vi "CalculateVIWiresLength.vi"(8 "error in (no error)":errorcluster, 11 "VI Refnum":refnum<vi>) -> (0 "error out":errorcluster, 2 "WiresDistance":i32, 3 "VI Refnum out":refnum<vi>)   [LabVIEW 2020]
uses:
  <vilib>/Utility/traverseref.llb/TRef TravTarget.ctl
  <vilib>/Utility/traverseref.llb/VI Scripting - Traverse.lvlib
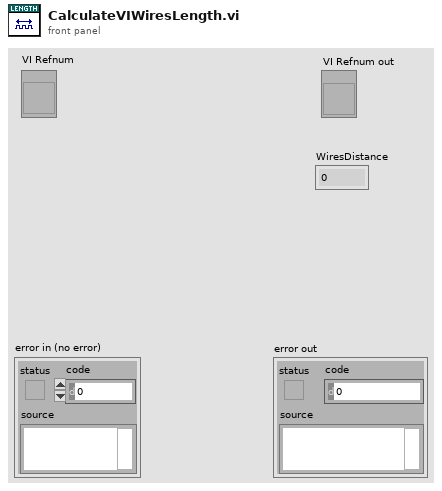
[diagram p1: front panel]
types:
  T1 = typedef "TRef TravTarget.ctl" = enum16{"FP", "BD", "Other"}
  T2 = cluster{"Position":cluster{"h":i16, "v":i16}, "Flags":i32, "Type":enum32{"LooseEnd", "Endpoint", "Bend", "Junction"}, "Up Joint Index":i16, "Down Joint Index":i16, "Left Joint Index":i16, "Right Joint Index":i16}[]
  T3 = cluster{"Position":cluster{"h":i16, "v":i16}, "Flags":i32, "Type":enum32{"LooseEnd", "Endpoint", "Bend", "Junction"}, "Up Joint Index":i16, "Down Joint Index":i16, "Left Joint Index":i16, "Right Joint Index":i16}
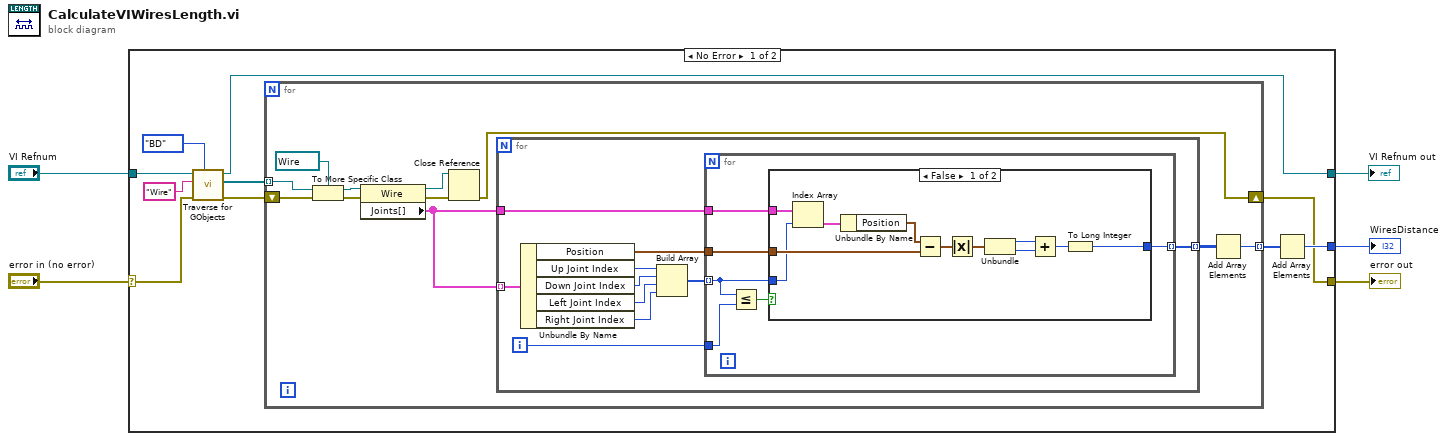
[diagram p0: block diagram]
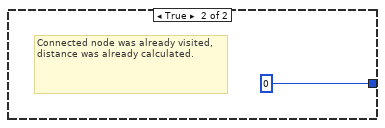
[diagram p2: hidden frame]
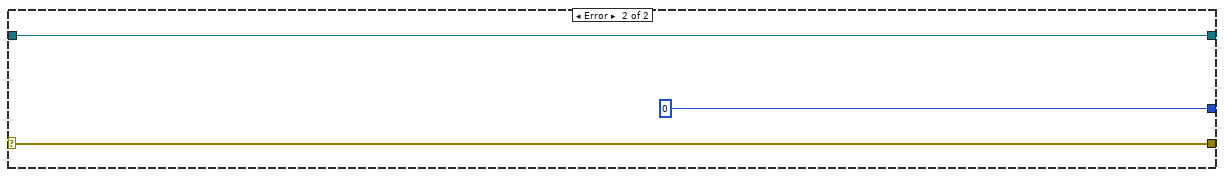
[diagram p3: hidden frame]
diagram:
  n1 = case shown="No Error" "error in (no error)" {
    selector: "error in (no error)" -> [w7 w57]
    tunnel: [w11 i16 0] -> w5
    tunnel: "VI Refnum" -> [w9 w55]
    tunnel: [w8 w57] -> w3
    tunnel: [w6 w55] -> w1
    frame No Error {
      n2 = call <vilib>:"Traverse for GObjects.vi"("Traverse Target"=TRef_TravTarget."BD", "error in (no error)"=w7, "Class Name"="Wire", "VI Refnum"=w9) -> ("error out"=w10:errorcluster, "References"=w13:refnum<vi>[], "dup VI Refnum"=w6:refnum<vi>)  [unwired: 4 in, 1 out]
      n3 = for {
        tunnel: w13 -> [w26] mode=indexing
        tunnel: [w21] -> w12 mode=indexing
        shift-right: [w17] -> w8
        shift-left: w10 -> [w20]
        n4 = To More Specific Class(target class=refnum<vi> refnum ("reference"), reference=w26, error in=w20) -> (specific class reference=w24:refnum<vi>, error out=w19:errorcluster)
        n5 = property class="Wire"(reference=w24, error in=w19) -> (reference out=w16:refnum<vi>, error out=w18:errorcluster, "Joints[]"=w23:T2)
        n6 = Close Reference(reference=w16, error in (no error)=w18) -> (error out=w17:errorcluster)
        n7 = for {
          tunnel: w23 -> [w32] mode=indexing
          tunnel: w23 -> [w31]
          tunnel: [w27] -> w22 mode=indexing
          i -> [w28]
          n8 = Unbundle By Name(w32) -> ("Position"=w29:cluster{"h":i16, "v":i16}, "Up Joint Index"=w36:i16, "Down Joint Index"=w35:i16, "Left Joint Index"=w34:i16, "Right Joint Index"=w33:i16)
          n9 = Build Array(w36, w35, w34, w33) -> (w30:i16[])
          n10 = for {
            tunnel: w31 -> [w42]
            tunnel: w30 -> [w38] mode=indexing
            tunnel: w29 -> [w41]
            tunnel: w28 -> [w40]
            tunnel: [w37] -> w27 mode=indexing
            n11 = Less Or Equal?(x=w38, y=w40) -> (x <= y?=w39:bool)
            n12 = case shown="False" w39 {
              tunnel: w42 -> [w53 _]
              tunnel: w41 -> [w50 _]
              tunnel: w38 -> [w44 _]
              tunnel: [w43 i16 0] -> w37
              frame False {
                n13 = Index Array(array=w53, index=w44) -> (element=w52:T3)
                n14 = Unbundle By Name(w52) -> ("Position"=w51:cluster{"h":i16, "v":i16})
                n15 = Subtract(x=w51, y=w50) -> (x-y=w49:cluster{"h":i16, "v":i16})
                n16 = Absolute Value(x=w49) -> (abs(x)=w48:cluster{"h":i16, "v":i16})
                n17 = Unbundle(w48) -> ("h"=w47:i16, "v"=w46:i16)
                n18 = Add(x=w47, y=w46) -> (x+y=w45:i16)
                n19 = To Long Integer(number=w45) -> (32bit integer=w43:i32)
              }
              frame True {
                # "Connected node was already visited, distance was already calculated."
              }
            }
          }
        }
        n20 = Add Array Elements(numeric array=w22) -> (sum=w21:i32)
      }
      n21 = Add Array Elements(numeric array=w12) -> (sum=w11:i32)
    }
    frame Error {
    }
  }
  "WiresDistance" <- w5
  "error out" <- w3
  "VI Refnum out" <- w1
